vi "h5_init_2D_v2.vi"(0 "files":path[](array[path]), 5 "RID":string, 7 "scan_config":T1={"v0 name"="radiant (nm)", "v0 num"=808, "v1 name"="none", "v1 num"=808, "scan_values"=[], "num rows"=808, "measurement"=0, "v0_config"={"hardware"=enum."radiant (nm)", "options"="", "repeats"=4, "loops"=1, "VISA"="COM9", "override_VISA"=TRUE}, "v1_config"={"hardware"=enum."radiant (nm)", "options"="", "repeats"=4, "loops"=1, "VISA"="COM9", "override_VISA"=TRUE}, "scope_config"={"VISA"="lecroy", "channels"=[enum."Channel 1"], "timeout (ms)"=100000, "max_points"=2500, "averages"=50, "noise filter"=enum."None"}} {"scope_config"."averages" min=1; "scope_config"."max_points" items=["50"=50, "100"=100, "250"=250, "500"=500, "1000"=1000, "2500"=2500, "5K"=5000, "10K"=10000, "25K"=25000, "50K"=50000, "100K"=100000, "250K"=250000, "500K"=500000, "1M"=1000000, "2M"=2000000, "2.5M"=2500000, "5M"=5000000, "10M"=10000000, "25M"=25000000, "50M"=50000000, "100M"=100000000]; "v1_config"."loops" min=1; "v1_config"."repeats" min=1; "v0_config"."loops" min=1; "v0_config"."repeats" min=1}, 11 "error in (no error)":errorcluster) -> (15 "error out":errorcluster)   [LabVIEW 2017, in "tools.lvlib"]
uses:
  tools.lvlib
  core/scan_config.ctl
  core/var_config.ctl
  ctrl/var_list.ctl
  hardware/lecroy/scope_config.ctl
  <vilib>/UPVI/lvhdf5/file.llb/LVH5F Operation.ctl
  <vilib>/UPVI/lvhdf5/attribute.llb/LVH5A Operation.ctl
  <vilib>/UPVI/lvhdf5/attribute.llb/Simple H5Awrite (Variant).vi
  <vilib>/UPVI/lvhdf5/attribute.llb/Simple H5Awrite.xnode
  <vilib>/UPVI/lvhdf5/library.llb/HDF5 Ref.ctl
  hardware/lecroy/lecroy.lvlib
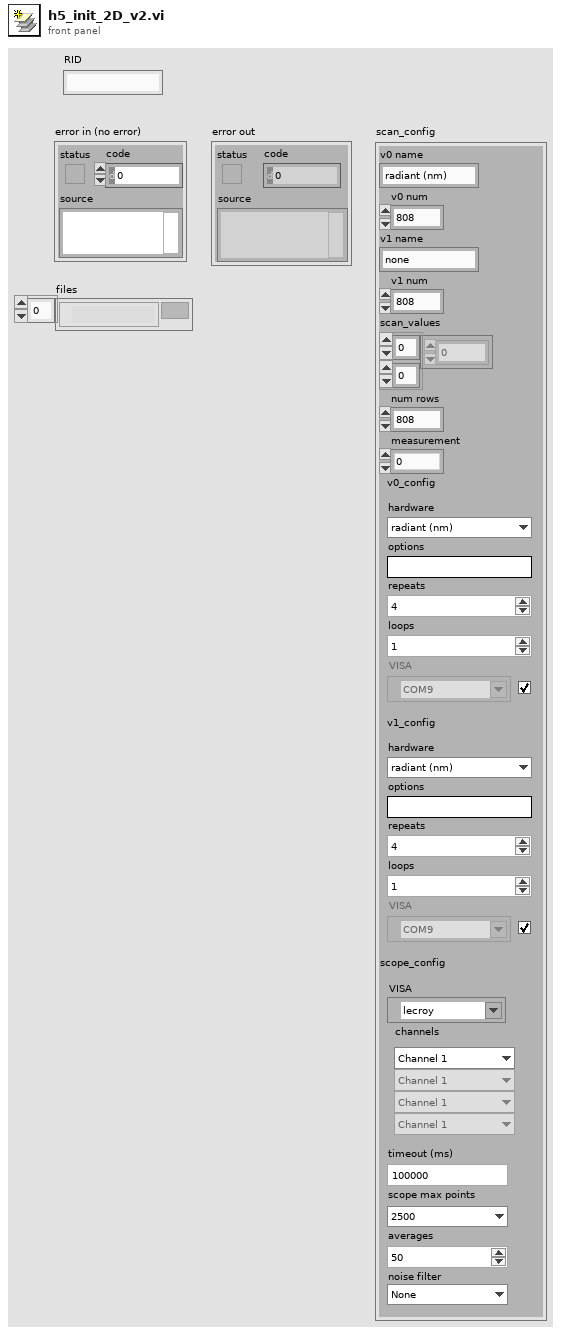
[diagram p1: front panel]
types:
  T1 = typedef "tools.lvlib/scan_config.ctl" = cluster{"v0 name":string, "v0 num":i32, "v1 name":string, "v1 num":i32, "scan_values":dbl[][], "num rows":i32, "measurement":i32, "v0_config":T2, "v1_config":T2, "scope_config":T4}
  T2 = typedef "tools.lvlib/var_config.ctl" = cluster{"hardware":T3, "options":string, "repeats":i32, "loops":i32, "VISA":refnum<visa-resource-name>, "override_VISA":bool}
  T3 = typedef "var_list.ctl" = enum16{"none", "AO voltage (V)", "delay (s)", "generic", "microwaves (GHz)", "radiant (nm)", "radiant thg (nm)", "sirah (nm)", "sirah_shg (nm)", "tenma voltage (V)", "wait (s)", "wf_freq (Hz)", "wf_amp (V)", "wf_amp_multi (V)", "wf_offset (V)", "wf_low_level (V)", "wf_high_level (V)", "wf_period (s)", "wf_pulse_width (s)", "wf_sample_rate (Sa/s)", "wf_multi_amp", "wf_multi_freq", "wf_arb_4chan", "WS7 setpoint (nm)"}
  T4 = typedef "lecroy.lvlib/scope_config.ctl" = cluster{"VISA":refnum<visa-resource-name>, "channels":enum16{"Channel 1", "Channel 2", "Channel 3", "Channel 4"}[], "timeout (ms)":u32, "max_points":i32, "averages":i32, "noise filter":enum16{"None", "+0.5 bit", "+1 bit", "+1.5 bits", "+2 bits", "+2.5 bits", "+3 bits"}}
  T5 = typedef "Semaphore RefNum" = refnum<k1>
  T6 = typedef "LVH5F Operation.ctl" = enum16{"open", "open or create", "create or replace", "create or replace (with confirmation)", "create", "open (read only)"}
  T7 = typedef "LVH5A Operation.ctl" = enum16{"open", "replace", "create", "open or create", "create or replace", "create or replace with confirmation"}
  T8 = typedef "HDF5 Ref.ctl" = refnum<k1>
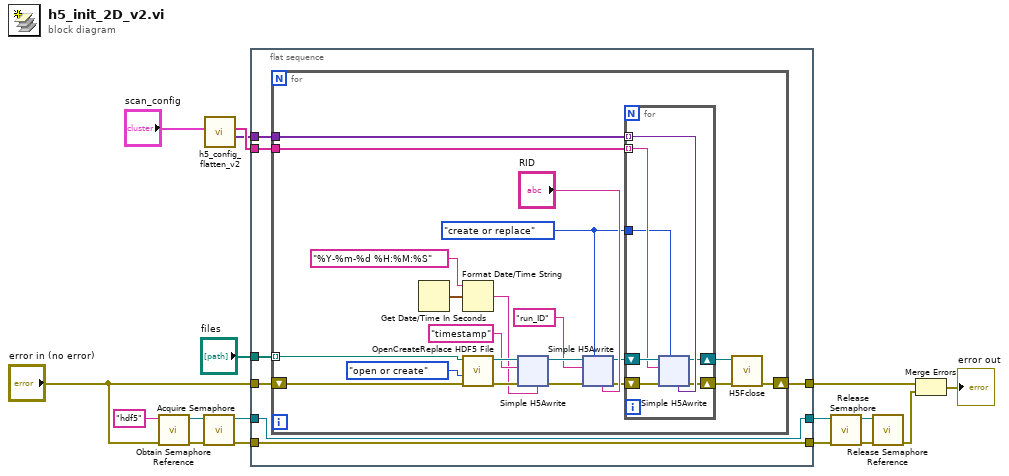
[diagram p0: block diagram]
diagram:
  n1 = call <vilib>:"Obtain Semaphore Reference.vi"("error in (no error)"="error in (no error)", "name (unnamed)"="hdf5") -> ("error out"=w16:errorcluster, "semaphore"=w17:T5)  [unwired: 3 in, 1 out]
  n2 = call <vilib>:"Acquire Semaphore.vi"("error in (no error)"=w16, "semaphore"=w17) -> ("error out"=w11:errorcluster, "semaphore out"=w10:T5)  [unwired: 3 in, 1 out]
  n3 = call "h5_config_flatten_v2.vi"("scan_config"="scan_config") -> ("Values out"=w1:variant[], "Names out"=w2:string[])  [unwired: 8 in, 1 out]
  n4 = flat-sequence {
    tunnel: "error in (no error)" -> [w21]
    tunnel: w11 -> [w24]
    tunnel: w10 -> [w23]
    tunnel: [w24] -> w9
    tunnel: [w23] -> w8
    tunnel: [w22] -> w7
    tunnel: "files" -> [w20]
    tunnel: w2 -> [w19]
    tunnel: w1 -> [w18]
    frame #0 {
      n5 = for {
        shift-right: [w34] -> w22
        shift-left: w21 -> [w33]
        tunnel: w20 -> [w32] mode=indexing
        tunnel: w19 -> [w29]
        tunnel: w18 -> [w28]
        w25 = LVH5A_Operation."create or replace" ("operation (create or replace)")
        n6 = Get Date/Time In Seconds() -> (seconds since 1Jan1904=w41:timestamp)
        n7 = Format Date/Time String(time format string (%c)="%Y-%m-%d %H:%M:%S", seconds (now)=w41) -> (date/time string=w40:string)  [unwired: 1 in]
        n8 = call <vilib>:"OpenCreateReplace HDF5 File.vi"("error in (no error)"=w33, "function (open or create)"=LVH5F_Operation."open or create", "path"=w32) -> ("error out"=w44:errorcluster, "HDF5 Ref out"=w45:T8)  [unwired: 5 in]
        n9 = xnode "Simple H5Awrite"("HDF5 Ref"=w45, "Name"="timestamp", "error in (no error)"=w44, "Value"=w40) -> ("HDF5 Ref out"=w38:T8, "error out"=w37:errorcluster)  [unwired: 1 in]
        n10 = xnode "Simple H5Awrite"("HDF5 Ref"=w38, "Name"="run_ID", "error in (no error)"=w37, "operation (open or create)"=w25, "Value"="RID") -> ("HDF5 Ref out"=w31:T8, "error out"=w30:errorcluster)
        n11 = for {
          tunnel: w29 -> [w51] mode=indexing
          tunnel: w28 -> [w50] mode=indexing
          shift-right: [w47] -> w27
          shift-left: w31 -> [w52]
          shift-right: [w48] -> w26
          shift-left: w30 -> [w49]
          tunnel: w25 -> [w46]
          n12 = xnode "Simple H5Awrite"("HDF5 Ref"=w52, "Name"=w51, "error in (no error)"=w49, "operation (open or create)"=w46, "Value"=w50) -> ("HDF5 Ref out"=w47:T8, "error out"=w48:errorcluster)
        }
        n13 = call <vilib>:"H5Fclose.vi"("error in (no error)"=w26, "HDF5 Ref"=w27) -> ("error out"=w34:errorcluster)  [unwired: 7 in]
      }
    }
  }
  n14 = call <vilib>:"Release Semaphore.vi"("error in (no error)"=w9, "semaphore"=w8) -> ("error out"=w14:errorcluster, "semaphore out"=w13:T5)  [unwired: 4 in]
  n15 = call <vilib>:"Release Semaphore Reference.vi"("error in (no error)"=w14, "semaphore"=w13) -> ("error out"=w6:errorcluster)  [unwired: 8 in, 1 out]
  n16 = Merge Errors(w7, w6) -> (→"error out":errorcluster)
